vi "real_web.vi"(11 "httpRequestID":u32) -> (3 "httpRequestID out":u32)   [LabVIEW 2011]
uses:
  <vilib>/addons/database/Connection.llb/DB Tools Open Connec (String).vi
  <vilib>/addons/database/Connection.llb/Conn Execute.vi
  <vilib>/addons/database/Recordset.llb/Rec Fetch Recordset Data (R).vi
  <vilib>/addons/database/Recordset.llb/Rec Destroy - Connection.vi
  <vilib>/addons/database/NI_Database_API.lvlib
  <vilib>/wsapi/NI_WebServices.lvlib
panel:
  out "error out":errorcluster
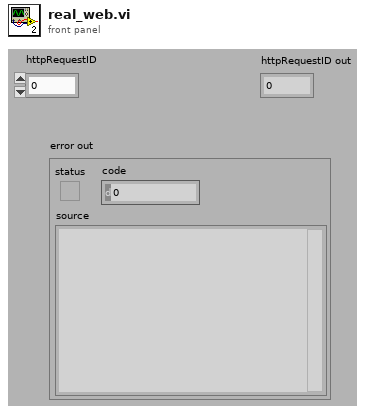
[diagram p1: front panel]
types:
  T1 = cluster{cluster{bool, bool, bool, bool}, cluster{bool, bool, bool, bool}, bool, bool, cluster{"value":string, "value":string}}
  T2 = typedef "NI_Database_API.lvlib/Conn ObjectReference.ctl" = refnum<k1>
  T3 = typedef "NI_Database_API.lvlib/Rec ObjectReference.ctl" = refnum<k1>
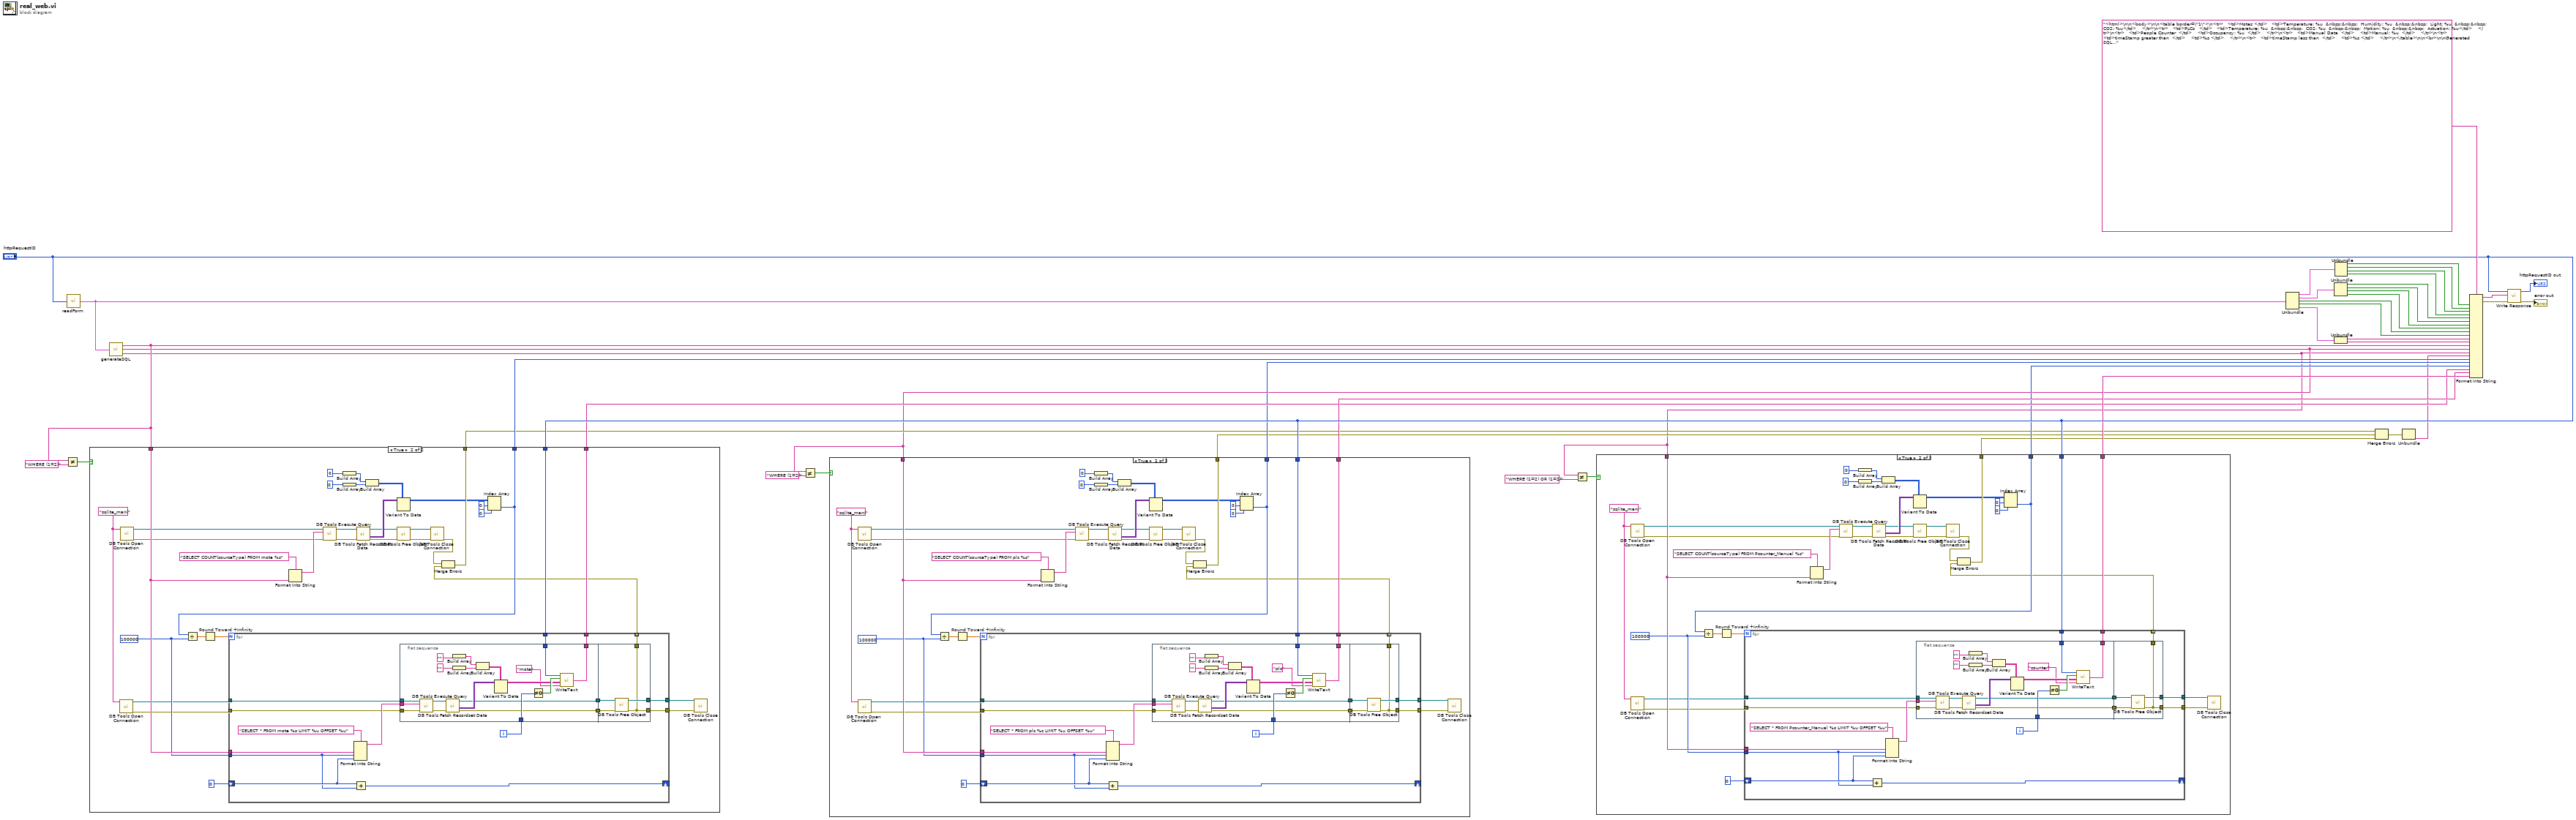
[diagram p0: block diagram]
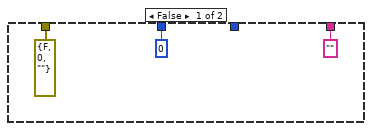
[diagram p2: hidden frame]
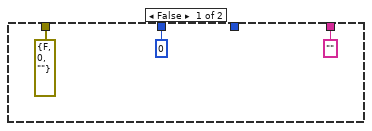
[diagram p3: hidden frame]
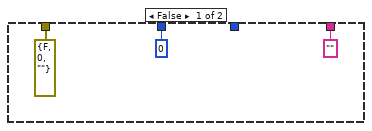
[diagram p4: hidden frame]
diagram:
  n1 = call "readForm.vi"("httpRequestID"="httpRequestID") -> ("output cluster"=w1:T1)
  n2 = call "generateSQL.vi"("input cluster"=w1) -> ("SQL command (mote)"=w10:string, "SQL command (plc)"=w6:string, "SQL command (counter and manual)"=w3:string)
  n3 = Not Equal?(x=w10, y="WHERE (1=2)") -> (x != y?=w8:bool)
  n4 = case shown="True" w8 {
    tunnel: w10 -> [_ w80]
    tunnel: "httpRequestID" -> [_ w79]
    tunnel: ["" ("hyperlink") w78] -> w19
    tunnel: [0 w77] -> w18
    tunnel: [errorcluster {"status"=FALSE, "code"=0, "source"=""} ("error IO") w76] -> w13
    frame False {
    }
    frame True {
      w48 = "sqlite_mani"
      w51 = u64 100000 ("y")
      n5 = call-poly <vilib>:"DB Tools Open Connection.vi"("connection information"=w48) -> ("error out"=w49:errorcluster, "connection reference"=w50:T2)  [unwired: 7 in]
      n6 = call-poly <vilib>:"DB Tools Open Connection.vi"("connection information"=w48) -> ("error out"=w46:errorcluster, "connection reference"=w47:T2)  [unwired: 7 in]
      n7 = Format Into String(format string="SELECT COUNT(sourceType) FROM mote %s", w80) -> (resulting string=w75:string)  [unwired: 2 in, 1 out]
      n8 = call-poly <vilib>:"DB Tools Execute Query.vi"("error in (no error)"=w46, "SQL query"=w75, "connection reference"=w47) -> ("error out"=w72:errorcluster, "recordset reference"=w73:T3)  [unwired: 5 in]
      n9 = Build Array(0) -> (w69:i32[])
      n10 = Build Array(0) -> (w70:i32[])
      n11 = call-poly <vilib>:"DB Tools Fetch Recordset Data.vi"("error in (no error)"=w72, "recordset reference"=w73) -> ("error out"=w59:errorcluster, "recordset data"=w68:variant[][], "recordset reference out"=w60:T3)  [unwired: 3 in]
      n12 = Build Array(w69, w70) -> (w71:i32[][])
      n13 = Variant To Data(type=w71, Variant=w68) -> (data=w63:i32[][])  [unwired: 1 in, 1 out]
      n14 = call-poly <vilib>:"DB Tools Free Object.vi"("error in (no error)"=w59, "recordset reference"=w60) -> ("error out"=w57:errorcluster, "connection reference"=w56:T2)  [unwired: 8 in]
      n15 = call <vilib>:"DB Tools Close Connection.vi"("error in (no error)"=w57, "connection reference"=w56) -> ("error out"=w55:errorcluster)  [unwired: 5 in]
      n16 = Index Array(array=w63, index (row)=0 ("index"), index (col)=0 ("disabled index (col)")) -> (element=w77:i32)
      n17 = Divide(x=w77, y=w51) -> (x/y=w61:dbl)
      n18 = Round Toward +Infinity(x=w61) -> (ceil(x): smallest int >= x=w58:dbl)
      n19 = for {
        N: w58 -> [_]
        tunnel: w50 -> [w94]
        tunnel: w49 -> [w93]
        tunnel: w80 -> [w92]
        shift-right: [w91] -> _
        shift-left: u64 0 -> [w90]
        tunnel: w51 -> [w89]
        tunnel: w79 -> [w87]
        tunnel: [w86] -> w78
        tunnel: [w83] -> w54
        tunnel: [w82] -> w53
        tunnel: [w81] -> w52 mode=indexing
        i -> [w88]
        n20 = Format Into String(format string="SELECT * FROM mote %s LIMIT %u OFFSET %u", w92, w89, w90) -> (resulting string=w95:string)  [unwired: 2 in, 1 out]
        n21 = Add(x=w90, y=w89) -> (x+y=w91:u64)
        n22 = flat-sequence {
          tunnel: w95 -> [w112]
          tunnel: w94 -> [w111]
          tunnel: w93 -> [w110]
          tunnel: w88 -> [w109]
          tunnel: w87 -> [w108]
          tunnel: [w107] -> w86
          tunnel: [w99] -> w85
          tunnel: [w98] -> w84
          tunnel: w85 -> [w119]
          tunnel: w84 -> [w118]
          tunnel: [w117] -> w83
          tunnel: [w116] -> w82
          tunnel: [w116] -> w81
          frame #0 {
            n23 = call-poly <vilib>:"DB Tools Execute Query.vi"("error in (no error)"=w110, "SQL query"=w112, "connection reference"=w111) -> ("error out"=w114:errorcluster, "recordset reference"=w113:T3)  [unwired: 5 in]
            n24 = call-poly <vilib>:"DB Tools Fetch Recordset Data.vi"("error in (no error)"=w114, "recordset reference"=w113) -> ("error out"=w98:errorcluster, "recordset data"=w115:variant[][], "recordset reference out"=w99:T3)  [unwired: 3 in]
            n25 = Build Array("") -> (w106:string[])
            n26 = Build Array("") -> (w105:string[])
            n27 = Build Array(w106, w105) -> (w104:string[][])
            n28 = Variant To Data(type=w104, Variant=w115) -> (data=w100:string[][])  [unwired: 1 in, 1 out]
            n29 = Not Equal To 0?(x=w109) -> (x != 0?=w101:bool)
            n30 = call "WriteText.vi"("filename"="mote", "Input data"=w100, "Append"=w101, "httpRequestID"=w108) -> ("hyperlink"=w107:string)
          }
          frame #1 {
            n31 = call-poly <vilib>:"DB Tools Free Object.vi"("error in (no error)"=w118, "recordset reference"=w119) -> ("error out"=w116:errorcluster, "connection reference"=w117:T2)  [unwired: 8 in]
          }
        }
      }
      n32 = Merge Errors(w55, w52) -> (w76:errorcluster)
      n33 = call <vilib>:"DB Tools Close Connection.vi"("error in (no error)"=w53, "connection reference"=w54) -> ()  [unwired: 5 in, 1 out]
    }
  }
  n34 = Not Equal?(x=w6, y="WHERE (1=2)") -> (x != y?=w7:bool)
  n35 = case shown="True" w7 {
    tunnel: w6 -> [_ w157]
    tunnel: "httpRequestID" -> [_ w156]
    tunnel: ["" ("hyperlink") w155] -> w20
    tunnel: [0 w154] -> w17
    tunnel: [errorcluster {"status"=FALSE, "code"=0, "source"=""} ("error IO") w153] -> w14
    frame False {
    }
    frame True {
      w128 = "sqlite_mani"
      w125 = u64 100000 ("y")
      n36 = call-poly <vilib>:"DB Tools Open Connection.vi"("connection information"=w128) -> ("error out"=w123:errorcluster, "connection reference"=w124:T2)  [unwired: 7 in]
      n37 = call-poly <vilib>:"DB Tools Open Connection.vi"("connection information"=w128) -> ("error out"=w127:errorcluster, "connection reference"=w126:T2)  [unwired: 7 in]
      n38 = Format Into String(format string="SELECT COUNT(sourceType) FROM plc %s", w157) -> (resulting string=w152:string)  [unwired: 2 in, 1 out]
      n39 = call-poly <vilib>:"DB Tools Execute Query.vi"("error in (no error)"=w127, "SQL query"=w152, "connection reference"=w126) -> ("error out"=w149:errorcluster, "recordset reference"=w150:T3)  [unwired: 5 in]
      n40 = Build Array(0) -> (w146:i32[])
      n41 = Build Array(0) -> (w147:i32[])
      n42 = call-poly <vilib>:"DB Tools Fetch Recordset Data.vi"("error in (no error)"=w149, "recordset reference"=w150) -> ("error out"=w136:errorcluster, "recordset data"=w145:variant[][], "recordset reference out"=w137:T3)  [unwired: 3 in]
      n43 = Build Array(w146, w147) -> (w148:i32[][])
      n44 = Variant To Data(type=w148, Variant=w145) -> (data=w140:i32[][])  [unwired: 1 in, 1 out]
      n45 = call-poly <vilib>:"DB Tools Free Object.vi"("error in (no error)"=w136, "recordset reference"=w137) -> ("error out"=w134:errorcluster, "connection reference"=w133:T2)  [unwired: 8 in]
      n46 = call <vilib>:"DB Tools Close Connection.vi"("error in (no error)"=w134, "connection reference"=w133) -> ("error out"=w132:errorcluster)  [unwired: 5 in]
      n47 = Index Array(array=w140, index (row)=0 ("index"), index (col)=0 ("disabled index (col)")) -> (element=w154:i32)
      n48 = Divide(x=w154, y=w125) -> (x/y=w138:dbl)
      n49 = Round Toward +Infinity(x=w138) -> (ceil(x): smallest int >= x=w135:dbl)
      n50 = for {
        N: w135 -> [_]
        tunnel: w124 -> [w171]
        tunnel: w123 -> [w170]
        tunnel: w157 -> [w169]
        shift-right: [w168] -> _
        shift-left: u64 0 -> [w167]
        tunnel: w125 -> [w166]
        tunnel: w156 -> [w164]
        tunnel: [w163] -> w155
        tunnel: [w160] -> w130
        tunnel: [w159] -> w129
        tunnel: [w158] -> w131 mode=indexing
        i -> [w165]
        n51 = Format Into String(format string="SELECT * FROM plc %s LIMIT %u OFFSET %u", w169, w166, w167) -> (resulting string=w172:string)  [unwired: 2 in, 1 out]
        n52 = Add(x=w167, y=w166) -> (x+y=w168:u64)
        n53 = flat-sequence {
          tunnel: w172 -> [w189]
          tunnel: w171 -> [w188]
          tunnel: w170 -> [w187]
          tunnel: w165 -> [w186]
          tunnel: w164 -> [w185]
          tunnel: [w184] -> w163
          tunnel: [w176] -> w162
          tunnel: [w175] -> w161
          tunnel: w162 -> [w196]
          tunnel: w161 -> [w195]
          tunnel: [w194] -> w160
          tunnel: [w193] -> w159
          tunnel: [w193] -> w158
          frame #0 {
            n54 = call-poly <vilib>:"DB Tools Execute Query.vi"("error in (no error)"=w187, "SQL query"=w189, "connection reference"=w188) -> ("error out"=w191:errorcluster, "recordset reference"=w190:T3)  [unwired: 5 in]
            n55 = call-poly <vilib>:"DB Tools Fetch Recordset Data.vi"("error in (no error)"=w191, "recordset reference"=w190) -> ("error out"=w175:errorcluster, "recordset data"=w192:variant[][], "recordset reference out"=w176:T3)  [unwired: 3 in]
            n56 = Build Array("") -> (w183:string[])
            n57 = Build Array("") -> (w182:string[])
            n58 = Build Array(w183, w182) -> (w181:string[][])
            n59 = Variant To Data(type=w181, Variant=w192) -> (data=w177:string[][])  [unwired: 1 in, 1 out]
            n60 = Not Equal To 0?(x=w186) -> (x != 0?=w178:bool)
            n61 = call "WriteText.vi"("filename"="plc", "Input data"=w177, "Append"=w178, "httpRequestID"=w185) -> ("hyperlink"=w184:string)
          }
          frame #1 {
            n62 = call-poly <vilib>:"DB Tools Free Object.vi"("error in (no error)"=w195, "recordset reference"=w196) -> ("error out"=w193:errorcluster, "connection reference"=w194:T2)  [unwired: 8 in]
          }
        }
      }
      n63 = Merge Errors(w132, w131) -> (w153:errorcluster)
      n64 = call <vilib>:"DB Tools Close Connection.vi"("error in (no error)"=w129, "connection reference"=w130) -> ()  [unwired: 5 in, 1 out]
    }
  }
  n65 = Not Equal?(x=w3, y="WHERE (1=2) OR (1=2)") -> (x != y?=w4:bool)
  n66 = case shown="True" w4 {
    tunnel: w3 -> [_ w234]
    tunnel: "httpRequestID" -> [_ w233]
    tunnel: ["" ("hyperlink") w232] -> w21
    tunnel: [0 w231] -> w16
    tunnel: [errorcluster {"status"=FALSE, "code"=0, "source"=""} ("error IO") w230] -> w15
    frame False {
    }
    frame True {
      w205 = "sqlite_mani"
      w204 = u64 100000 ("y")
      n67 = call-poly <vilib>:"DB Tools Open Connection.vi"("connection information"=w205) -> ("error out"=w202:errorcluster, "connection reference"=w203:T2)  [unwired: 7 in]
      n68 = call-poly <vilib>:"DB Tools Open Connection.vi"("connection information"=w205) -> ("error out"=w200:errorcluster, "connection reference"=w201:T2)  [unwired: 7 in]
      n69 = Format Into String(format string="SELECT COUNT(sourceType) FROM Pcounter_Manual %s", w234) -> (resulting string=w229:string)  [unwired: 2 in, 1 out]
      n70 = call-poly <vilib>:"DB Tools Execute Query.vi"("error in (no error)"=w200, "SQL query"=w229, "connection reference"=w201) -> ("error out"=w226:errorcluster, "recordset reference"=w227:T3)  [unwired: 5 in]
      n71 = Build Array(0) -> (w223:i32[])
      n72 = Build Array(0) -> (w224:i32[])
      n73 = call-poly <vilib>:"DB Tools Fetch Recordset Data.vi"("error in (no error)"=w226, "recordset reference"=w227) -> ("error out"=w213:errorcluster, "recordset data"=w222:variant[][], "recordset reference out"=w214:T3)  [unwired: 3 in]
      n74 = Build Array(w223, w224) -> (w225:i32[][])
      n75 = Variant To Data(type=w225, Variant=w222) -> (data=w217:i32[][])  [unwired: 1 in, 1 out]
      n76 = call-poly <vilib>:"DB Tools Free Object.vi"("error in (no error)"=w213, "recordset reference"=w214) -> ("error out"=w211:errorcluster, "connection reference"=w210:T2)  [unwired: 8 in]
      n77 = call <vilib>:"DB Tools Close Connection.vi"("error in (no error)"=w211, "connection reference"=w210) -> ("error out"=w209:errorcluster)  [unwired: 5 in]
      n78 = Index Array(array=w217, index (row)=0 ("index"), index (col)=0 ("disabled index (col)")) -> (element=w231:i32)
      n79 = Divide(x=w231, y=w204) -> (x/y=w215:dbl)
      n80 = Round Toward +Infinity(x=w215) -> (ceil(x): smallest int >= x=w212:dbl)
      n81 = for {
        N: w212 -> [_]
        tunnel: w203 -> [w248]
        tunnel: w202 -> [w247]
        tunnel: w234 -> [w246]
        shift-right: [w245] -> _
        shift-left: u64 0 -> [w244]
        tunnel: w204 -> [w243]
        tunnel: w233 -> [w241]
        tunnel: [w240] -> w232
        tunnel: [w237] -> w207
        tunnel: [w236] -> w206
        tunnel: [w235] -> w208 mode=indexing
        i -> [w242]
        n82 = Add(x=w244, y=w243) -> (x+y=w245:u64)
        n83 = Format Into String(format string="SELECT * FROM Pcounter_Manual %s LIMIT %u OFFSET %u", w246, w243, w244) -> (resulting string=w249:string)  [unwired: 2 in, 1 out]
        n84 = flat-sequence {
          tunnel: w249 -> [w266]
          tunnel: w248 -> [w265]
          tunnel: w247 -> [w264]
          tunnel: w242 -> [w263]
          tunnel: w241 -> [w262]
          tunnel: [w261] -> w240
          tunnel: [w253] -> w239
          tunnel: [w252] -> w238
          tunnel: w239 -> [w273]
          tunnel: w238 -> [w272]
          tunnel: [w271] -> w237
          tunnel: [w270] -> w236
          tunnel: [w270] -> w235
          frame #0 {
            n85 = call-poly <vilib>:"DB Tools Execute Query.vi"("error in (no error)"=w264, "SQL query"=w266, "connection reference"=w265) -> ("error out"=w268:errorcluster, "recordset reference"=w267:T3)  [unwired: 5 in]
            n86 = call-poly <vilib>:"DB Tools Fetch Recordset Data.vi"("error in (no error)"=w268, "recordset reference"=w267) -> ("error out"=w252:errorcluster, "recordset data"=w269:variant[][], "recordset reference out"=w253:T3)  [unwired: 3 in]
            n87 = Build Array("") -> (w260:string[])
            n88 = Build Array("") -> (w259:string[])
            n89 = Build Array(w260, w259) -> (w258:string[][])
            n90 = Variant To Data(type=w258, Variant=w269) -> (data=w254:string[][])  [unwired: 1 in, 1 out]
            n91 = Not Equal To 0?(x=w263) -> (x != 0?=w255:bool)
            n92 = call "WriteText.vi"("filename"="counter", "Input data"=w254, "Append"=w255, "httpRequestID"=w262) -> ("hyperlink"=w261:string)
          }
          frame #1 {
            n93 = call-poly <vilib>:"DB Tools Free Object.vi"("error in (no error)"=w272, "recordset reference"=w273) -> ("error out"=w270:errorcluster, "connection reference"=w271:T2)  [unwired: 8 in]
          }
        }
      }
      n94 = Merge Errors(w209, w208) -> (w230:errorcluster)
      n95 = call <vilib>:"DB Tools Close Connection.vi"("error in (no error)"=w206, "connection reference"=w207) -> ()  [unwired: 5 in, 1 out]
    }
  }
  n96 = Unbundle(w1) -> (w37:cluster{bool, bool, bool, bool}, w36:cluster{bool, bool, bool, bool}, w27:bool, w26:bool, w25:cluster{"value":string, "value":string})
  n97 = Unbundle(w36) -> (w31:bool, w30:bool, w29:bool, w28:bool)
  n98 = Unbundle(w25) -> ("value"=w24:string, "value"=w23:string)
  n99 = Unbundle(w37) -> (w35:bool, w34:bool, w33:bool, w32:bool)
  n100 = Merge Errors(w13, w14, w15) -> (w12:errorcluster)
  n101 = Unbundle(w12) -> ("source"=w11:string)  [unwired: 2 out]
  n102 = Format Into String(format string="<html>\n\n<body>\n\n<table border=\"1\">\n<tr>   <td>Motes </td>   <td>Temperature: %u  &nbsp;&nbsp;  Humidity: %u  &nbsp;&nbsp;  Light: %u  &nbsp;&nbsp;  CO2: %u</td>    </tr>\n<tr>   <td>PLCs   </td>   <td>Temperature: %u  &nbsp;&nbsp;  CO2: %u  &nbsp;&nbsp;  Motion: %u  &nbsp;&nbsp;  Actuation: %u</td>    </tr>\n<tr>   <td>People Counter  </td>    <td>Occupancy: %u  </td>    </tr>\n<tr>   <td>Manual Data  </td>    <td>Manual: %u  </td>    </tr>\n<tr>   <td>timeStamp greater than  </td>    <td>%s </td>    </tr>\n<tr>   <td>timeStamp less than  </td>    <td>%s </td>    </tr>\n</table>\n\n<br>\n\nGenerated SQL command (mote table): %s  <br>\nGenerated SQL command (plc table): %s  <br>\nGenerated SQL command (counter and manual tables): %s  <br> <br>\n\nAccess to database msg:  %s  <br> <br>\n\n(Number of retrieved records) <br>\nmote table: %u <br>\nplc table: %u <br>\ncounter and manual table: %u <br> <br>\n\n%s <br>\n%s <br>\n%s <br>\n\n</body>\n\n</html>", w35, w34, w33, w32, w31, w30, w29, w28, w27, w26, w24, w23, w10, w6, w3, w11, w18, w17, w16, w19, w20, w21) -> (resulting string=w42:string, error out=w41:errorcluster)  [unwired: 2 in]
  n103 = call <vilib>:"Write Response.vi"("error in (no error)"=w41, "response string"=w42, "httpRequestID"="httpRequestID") -> ("error out"=→"error out":errorcluster, "httpRequestID out"=→"httpRequestID out":u32)  [unwired: 7 out]
